vi "Mode 3.vi"() -> ()   [LabVIEW 2020]
uses:
  <vilib>/MakerHub/LINX/Private/Device/Type Defs/Pulse Polarity.ctl
  <vilib>/Platform/TimedLoop/XDataNode/timing_clust.ctl
  <vilib>/Platform/TimedLoop/XDataNode/nitl_modes.ctl
  <vilib>/Platform/TimedLoop/XDataNode/wakeup.ctl
  <vilib>/MakerHub/LINX/Public/Peripherals/Digital/Digital Write N Chans.vi
  <vilib>/MakerHub/LINX/Public/Peripherals/Digital/Digital Read N Chans.vi
  <vilib>/MakerHub/LINX/Public/Peripherals/PWM/PWM Set Duty Cycle 1 Chan.vi
  <vilib>/MakerHub/LINX/Private/Local IO/LinxDigitalWrite.vi
  <vilib>/MakerHub/LINX/Public/Utilities/Check Channel.vi
  <vilib>/MakerHub/LINX/Private/Local IO/LinxDigitalRead.vi
  <vilib>/MakerHub/LINX/Public/Utilities/Open Serial.vi
  <vilib>/MakerHub/LINX/Private/Utilties/Generate Error.vi
  <vilib>/MakerHub/LINX/Public/Sensors/Motion/Servo/Servo Open N Channels.vi
  <vilib>/MakerHub/LINX/Public/Sensors/Motion/Servo/Servo Set Pulse Width One Channel.vi
  <vilib>/MakerHub/LINX/Public/Peripherals/PWM/PWM Set Duty Cycle N Chans.vi
  <vilib>/MakerHub/LINX/Public/Sensors/Motion/Servo/Servo Close N Channels.vi
  <vilib>/platform/TimedLoop/XDataNode/XDataNode.xnode
  <vilib>/MakerHub/LINX/LMH-LINX.lvlib
  <vilib>/Platform/TimedLoop/XDataNode/XDNodeRunTimeDep.lvlib
  <vilib>/MakerHub/LINX/Public/Sensors/Motion/Servo/Servo.lvlib
  <vilib>/MakerHub/LINX/Private/Device/Device.lvlib
panel:
  in  "Titik Stop":u16=115
  in  "Color Check?":bool
  out "Blue Freq":u32
  out "Green Freq":u32
  out "Red Freq":u32
  out "Blue Workpiece":bool
  in  "Values":bool[](array[boolean])
  in  "Servo Slider 2 Angle":u16(knob)=82 scale=0.0..180.0
  in  "Servo Slider 1 Angle":u16(knob)=84 scale=0.0..180.0
  in  "Servo Magazine Angle":u16(knob)=115 scale=0.0..180.0
  in  "Servo Slider 2":u8=4
  in  "Servo Slider 1":u8=5
  in  "Servo Magazine":u8=3
  in  "Slider Counter":dbl[](array[numeric])=[0.0, 0.0, 0.0, 13.0]
  out "Green Workpiece":bool
  out "Red Workpiece":bool
  in  "Main Program":T1(array[cluster])=[{"Mode"=enum."Idle", "Limit"=enum."Tidak Ada", "Delay"=1000, "Point"=0, "Row"=0}, {"Mode"=enum."Cek Ketersediaan", "Limit"=enum."Tidak Ada", "Delay"=500, "Point"=0, "Row"=1}, {"Mode"=enum."Workpiece Masuk", "Limit"=enum."Tidak Ada", "Delay"=0, "Point"=0, "Row"=2}, {"Mode"=enum."Cek Warna", "Limit"=enum."Tidak Ada", "Delay"=1000, "Point"=0, "Row"=3}, {"Mode"=enum."Cek Counter", "Limit"=enum."Tidak Ada", "Delay"=1000, "Point"=0, "Row"=4}, {"Mode"=enum."Servo Set", "Limit"=enum."Tidak Ada", "Delay"=1000, "Point"=0, "Row"=5}, {"Mode"=enum."Conveyor Jalan", "Limit"=enum."Tidak Ada", "Delay"=0, "Point"=0, "Row"=6}, {"Mode"=enum."Servo Reset", "Limit"=enum."Tidak Ada", "Delay"=1000, "Point"=0, "Row"=7}, {"Mode"=enum."Counter", "Limit"=enum."Tidak Ada", "Delay"=0, "Point"=0, "Row"=8}, {"Mode"=enum."Go To", "Limit"=enum."Tidak Ada", "Delay"=0, "Point"=1, "Row"=9}]
  in  "Stop Main Program":bool
  out "Row":i32
  in  "Start Main Program":bool
  in  "Check Point":i32
  in  "STOP":bool
  in  "Speed Pin":u8=2
  in  "Sensors Pin":u8[](array[numeric])=[30, 34, 36, 38, 36, 38]
  out "Sensor Value":bool[](array[boolean])
  in  "Duty Cycle":dbl(knob) scale=0.0..100.0
  out "Device Name":string
  in  "Arduino Port":refnum<visa-resource-name>="N/A"
  # "LOW COST MPS SORTING BASED ARDUINO"
  # "MAIN PROGRAM"
  # "PROJECT MONITOR"
  # "Slider 1"
  # "Slider 2"
  # "Slider 3"
  # "INPUT/OUTPUT CONTROL"
  # "Index Array Sensors Pin\n\n0. IR Sensor Stock Check\n1. IR Sensor Slider 1\n2. IR Sensor Slider 2\n3. IR Sensor Slider 3"
  # "Mechatronics Engineering 2nd Generation - Vocational High School 2 Bojonegoro"
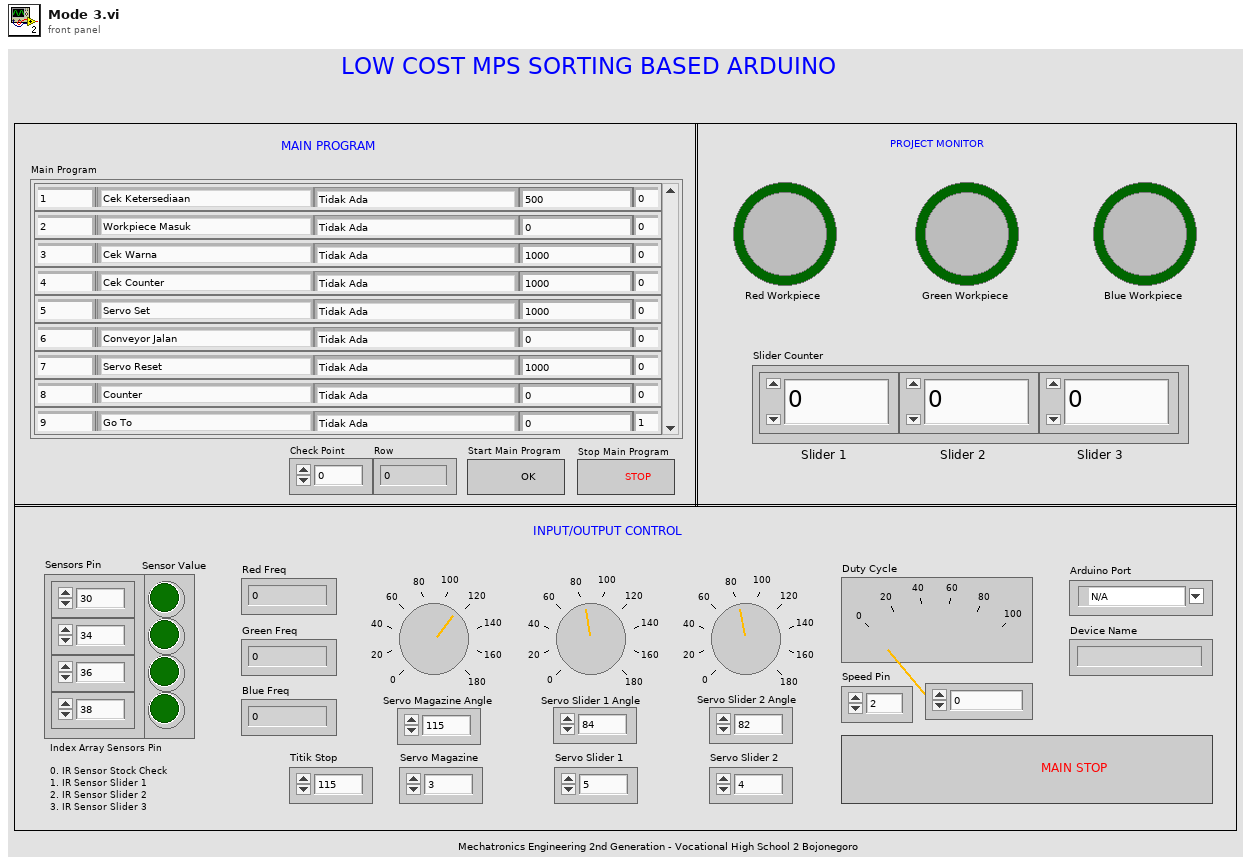
[diagram p1: front panel]
types:
  T1 = cluster{"Mode":enum16{"Idle", "Cek Ketersediaan", "Workpiece Masuk", "Cek Warna", "Servo Set", "Conveyor Jalan", "Servo Reset", "Counter", "Cek Counter", "Go To"}, "Limit":enum16{"Tidak Ada", "Sensor Slider"}, "Delay":i32, "Point":i32, "Row":i32}[]
  T2 = typedef "XDNodeRunTimeDep.lvlib/timing_clust.ctl" = cluster{"Expected End [f-1]":u64, "Actual End [f-1]":u64, "Finished Late? [f-1]":bool, "Expected End [i-1]":u64, "Actual End [i-1]":u64, "Finished Late? [i-1]":bool, "Expected Start [i]":u64, "Actual Start [i]":u64, "Expected Start [f]":u64, "Actual Start [f]":u64, "Source Name":string, "Structure Name":string, "Period":i64, "Deadline":i64, "Offset":i64, "Start":i64, "Priority":i32, "Timeout":i32, "Mode":T3, "Wakeup Reason":T4, "Error":errorcluster, "Source Type":string, "Secondary Source Type":string, "Global End Time":u64, "Global Start Time":u64, "Frame Duration":u64, "Iteration Duration":u64, "Assigned CPU":i32, "I/O Scan Engine Mode":u32}
  T3 = typedef "XDNodeRunTimeDep.lvlib/nitl_modes.ctl" = enum32{"No Change", "Process missed periods, maintain original phase", "Discard missed periods, maintain original phase", "Process missed periods, ignore original phase", "Discard missed periods, ignore original phase"}
  T4 = typedef "XDNodeRunTimeDep.lvlib/wakeup.ctl" = enum32{"Normal", "Aborted", "Asynchronous wakeup", "Timing source error", "Timed loop error", "Timeout"}
  T5 = cluster{"Mode":enum16{"Idle", "Cek Ketersediaan", "Workpiece Masuk", "Cek Warna", "Servo Set", "Conveyor Jalan", "Servo Reset", "Counter", "Cek Counter", "Go To"}, "Limit":enum16{"Tidak Ada", "Sensor Slider"}, "Delay":i32, "Point":i32, "Row":i32}
  T6 = enum16{"Idle", "Cek Ketersediaan", "Workpiece Masuk", "Cek Warna", "Servo Set", "Conveyor Jalan", "Servo Reset", "Counter", "Cek Counter", "Go To"}
  T7 = typedef "LMH-LINX.lvlib/LINX Ref.ctl" = cluster{"IO":T8, "Interface":T9, "LINX Device Config":T10}
  T8 = typedef "LMH-LINX.lvlib/Platform.ctl" = enum16{"Remote", "Local"}
  T9 = typedef "LMH-LINX.lvlib/Interface.ctl" = enum16{"Serial", "TCP"}
  T10 = typedef "LMH-LINX.lvlib/Device.lvlib/LINX Device Config.ctl" = cluster{"Interface":T9, "COM Port":refnum<visa-resource-name>, "TCP Configuration":T11, "Device Family":u8, "Device ID":u8, "Device Name":string, "TCP Ref":refnum<k5>, "Channels":T12}
  T11 = typedef "LMH-LINX.lvlib/Device.lvlib/TCP Config.ctl" = cluster{"IP Address":string, "Port":u16}
  T12 = typedef "LMH-LINX.lvlib/Channels.ctl" = cluster{"DI":u8[], "DO":u8[], "AI":u8[], "AO":u8[], "PWM":u8[], "QE":u8[], "UART":u8[], "I2C 2":u8[], "SPI":u8[], "CAN":u8[], "Servo":u8[], "AI Ref (V)":dbl, "AI Resolution (Bits)":u8, "AO Ref (V)":dbl, "AO Resolution (Bits)":u8}
  T13 = typedef "LMH-LINX.lvlib/Device.lvlib/Pulse Polarity.ctl" = enum8{"Active Low", "Active High"}
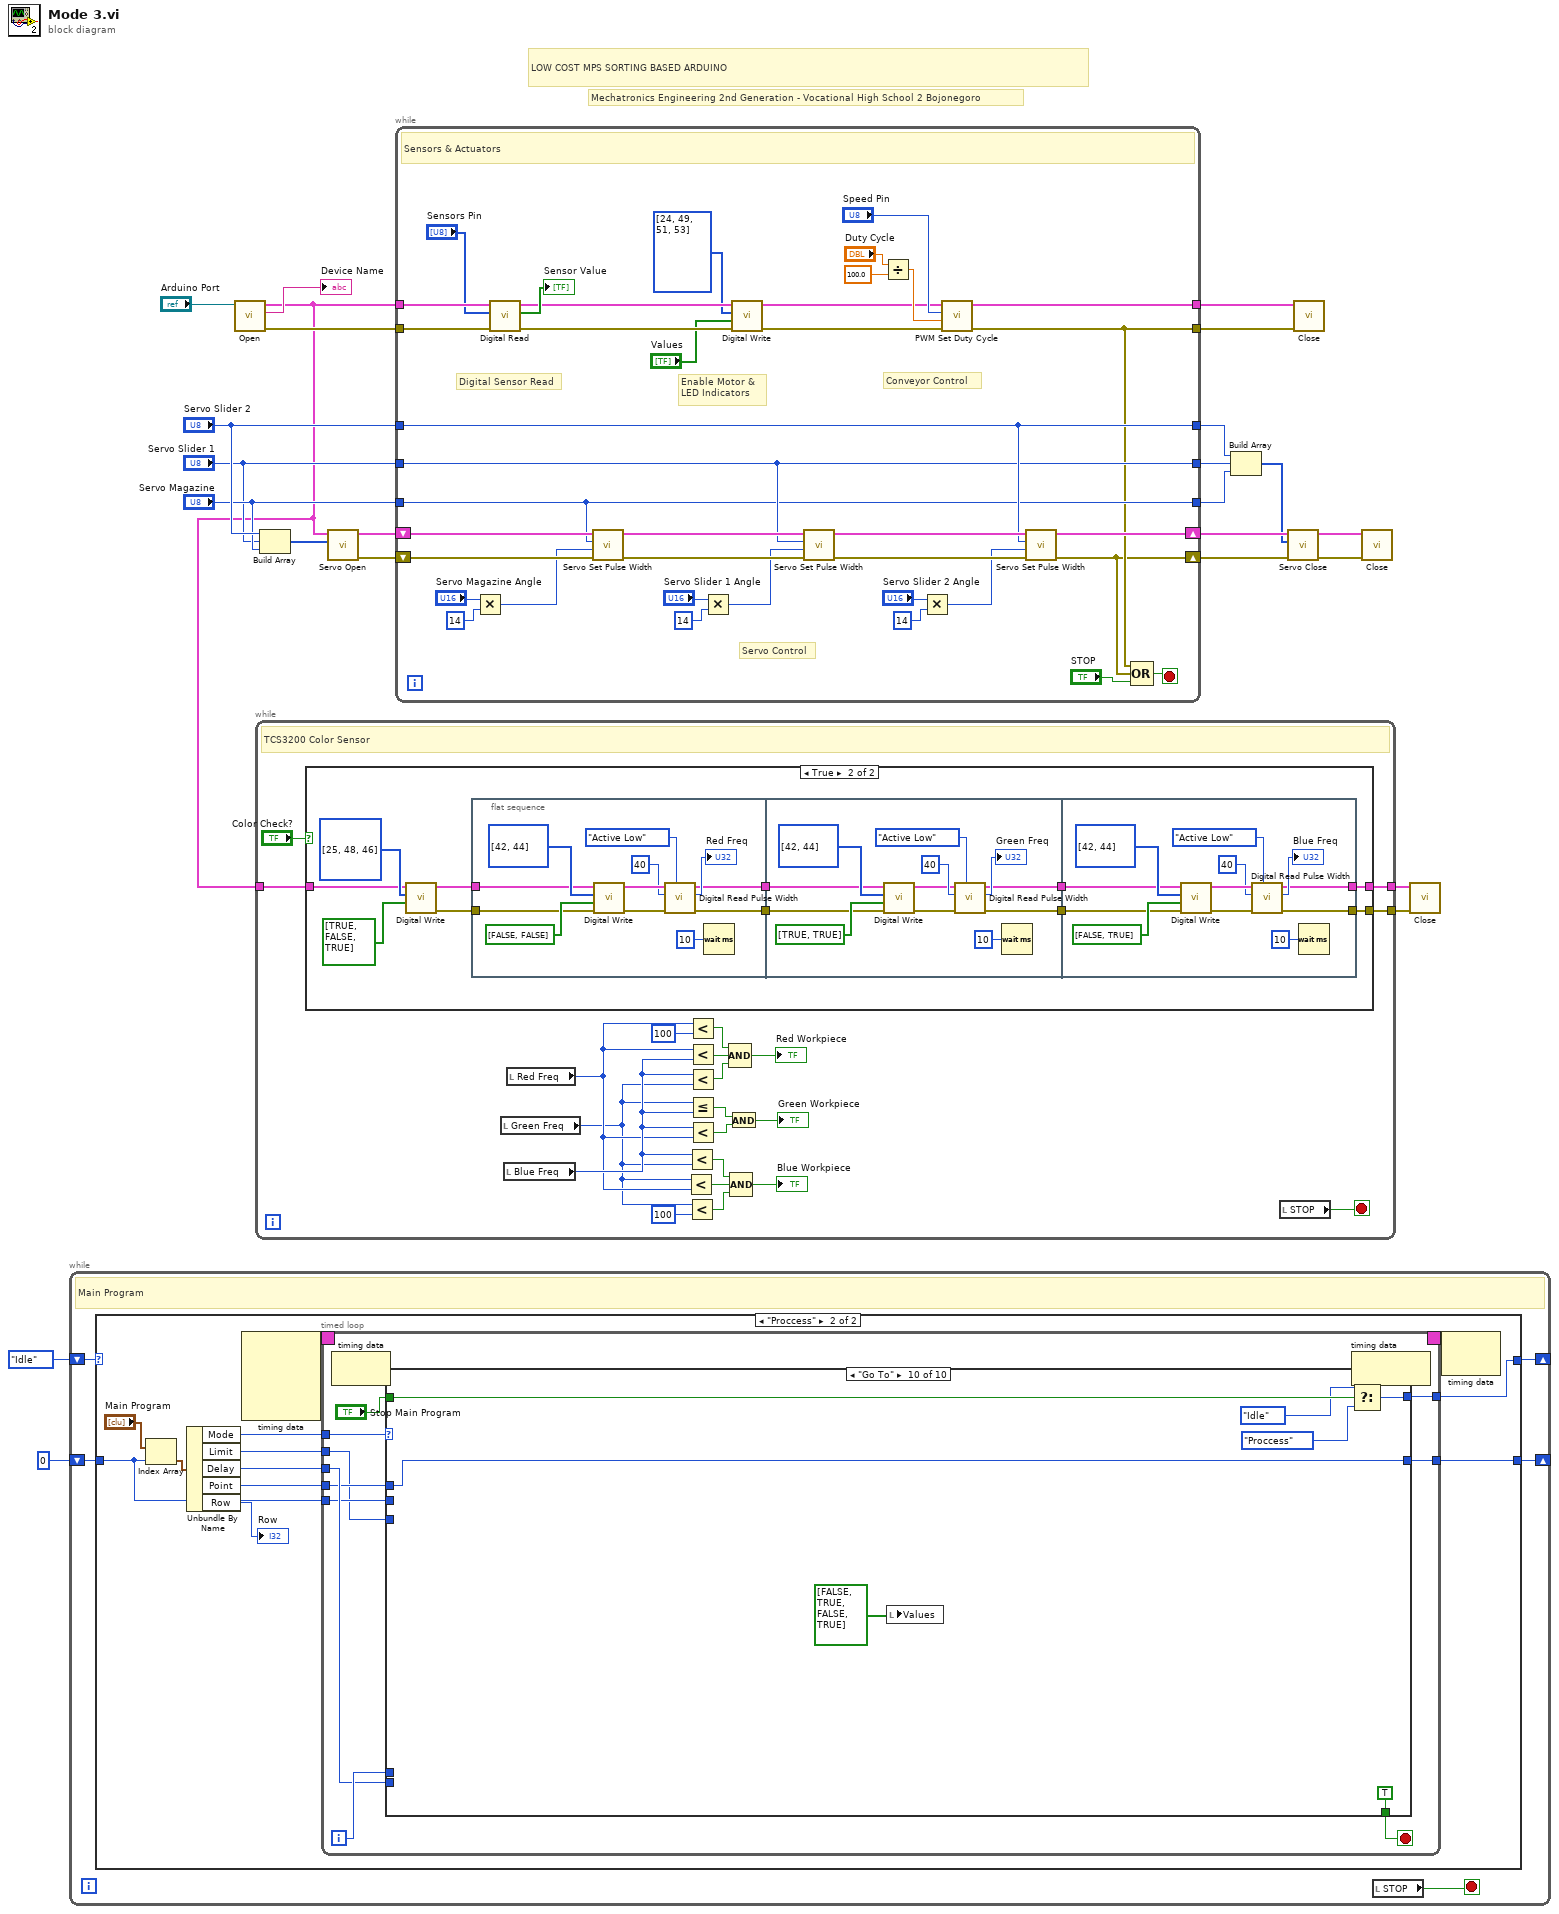
[diagram p0: block diagram]
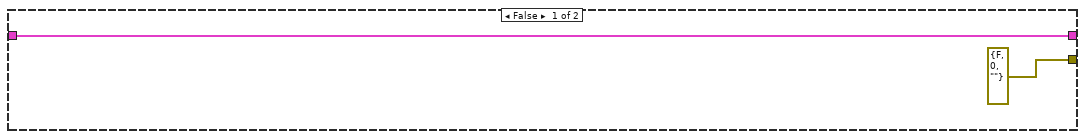
[diagram p2: hidden frame]
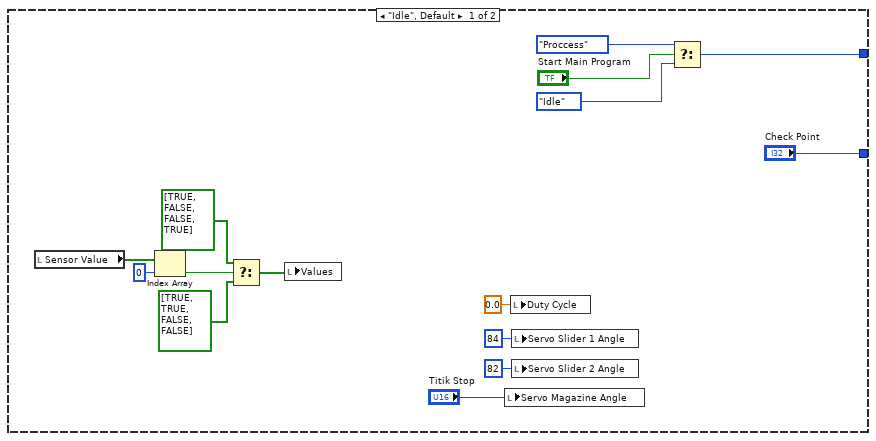
[diagram p3: hidden frame]
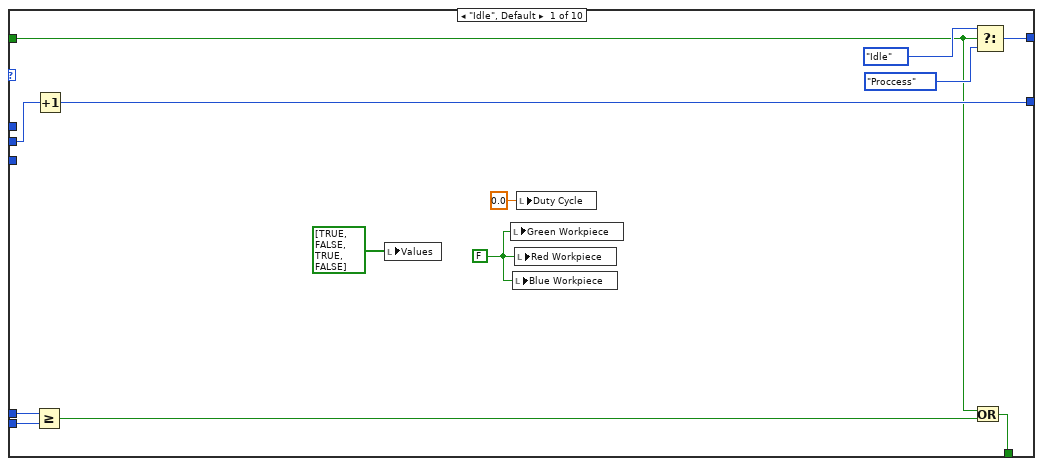
[diagram p4: hidden frame]
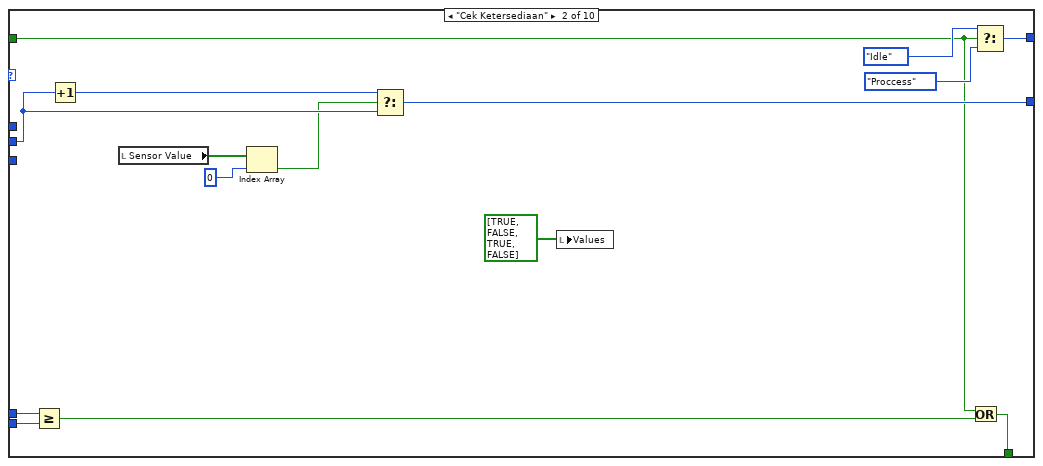
[diagram p5: hidden frame]
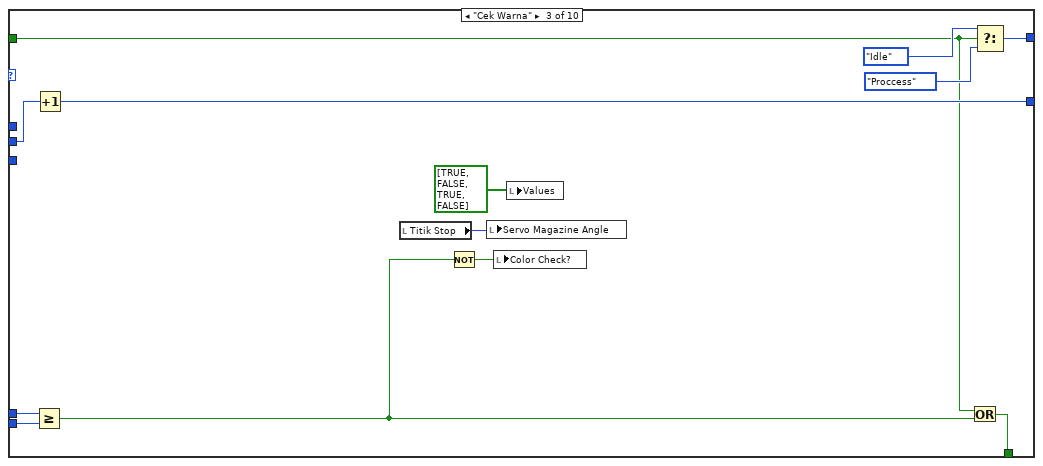
[diagram p6: hidden frame]
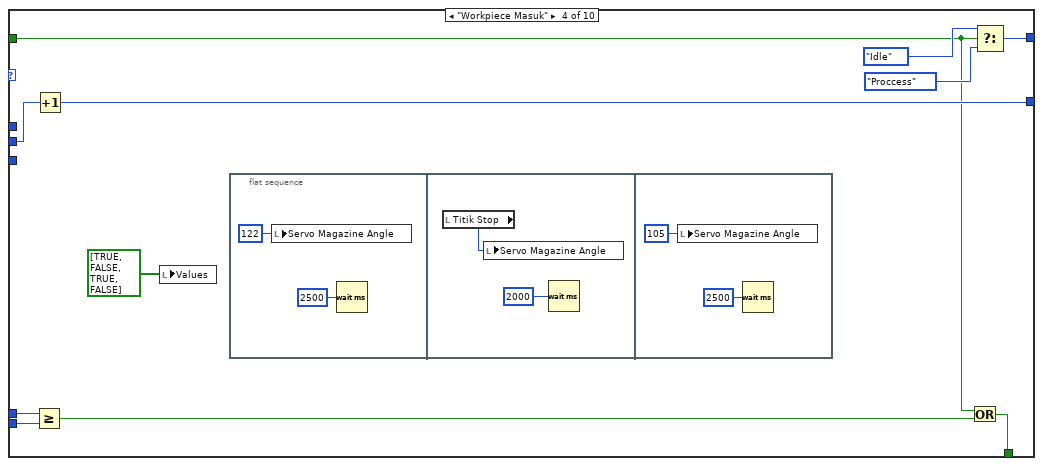
[diagram p7: hidden frame]
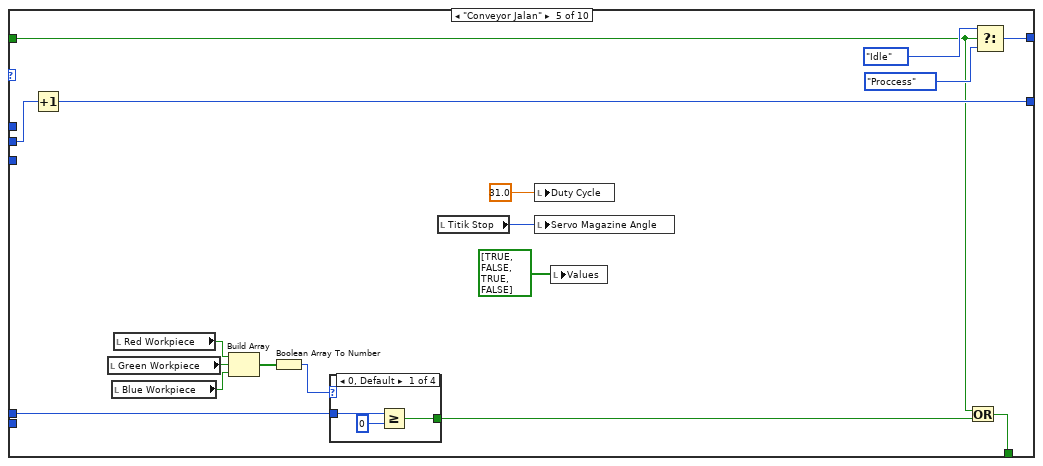
[diagram p8: hidden frame]
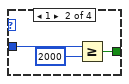
[diagram p9: hidden frame]
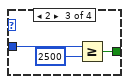
[diagram p10: hidden frame]
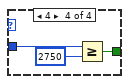
[diagram p11: hidden frame]
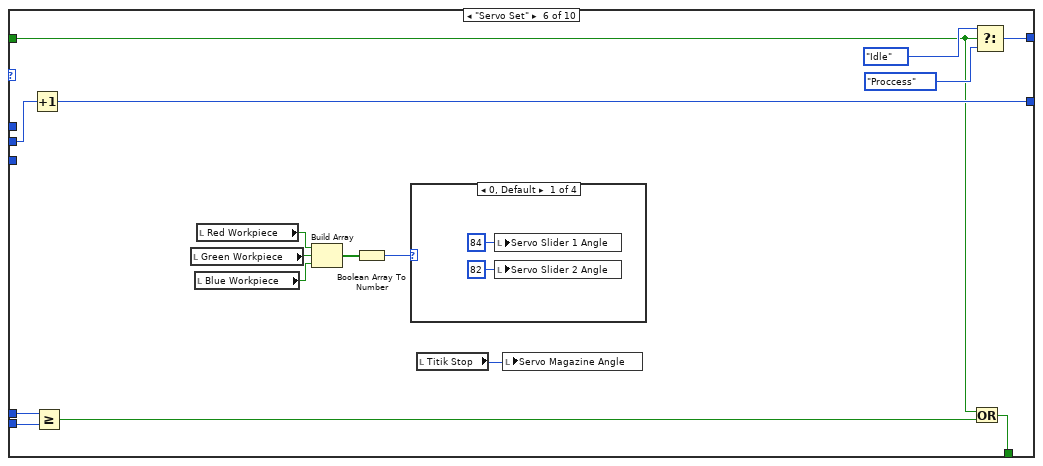
[diagram p12: hidden frame]
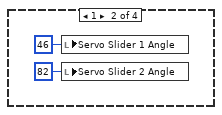
[diagram p13: hidden frame]
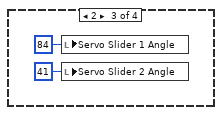
[diagram p14: hidden frame]
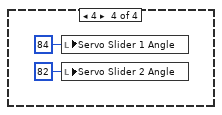
[diagram p15: hidden frame]
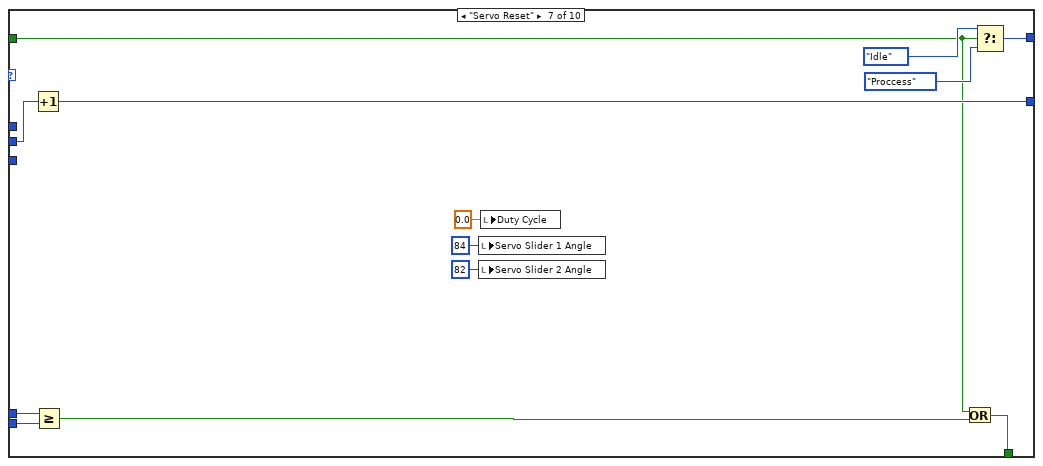
[diagram p16: hidden frame]
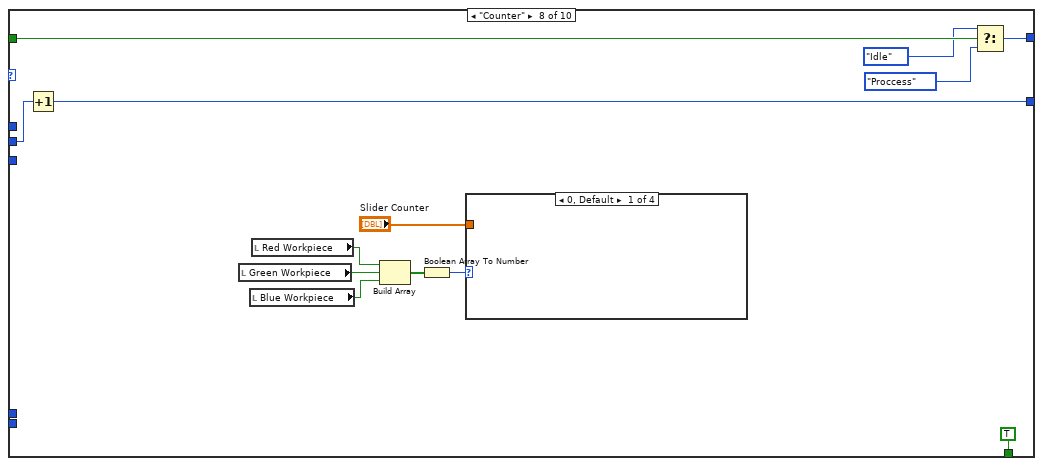
[diagram p17: hidden frame]
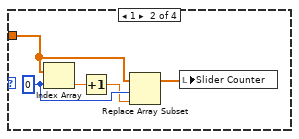
[diagram p18: hidden frame]
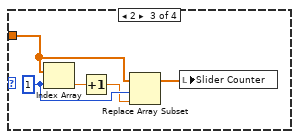
[diagram p19: hidden frame]
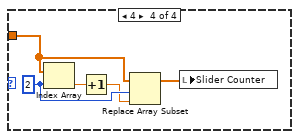
[diagram p20: hidden frame]
diagram:
  # "Mechatronics Engineering 2nd Generation - Vocational High School 2 Bojonegoro"
  # "LOW COST MPS SORTING BASED ARDUINO"
  n1 = while {
    shift-right: [w27] -> _
    shift-left: enum16{"Idle", "Proccess"}."Idle" -> [w28]
    shift-right: [w25] -> _
    shift-left: 0 ("index") -> [w26]
    stop <- w29 stop-if-true
    # "Main Program"
    n2 = case shown="\"Proccess\"" w28 {
      tunnel: [w44 w53] -> w27
      tunnel: w26 -> [_ w52]
      tunnel: ["Check Point" w51] -> w25
      frame "Idle", Default {
        n3 = local read "Sensor Value"() -> (w36:bool[])
        n4 = Index Array(array=w36, index=0) -> (element=w34:bool)
        n5 = Select(t=bool[] [TRUE, FALSE, FALSE, TRUE] ("Values"), s=w34, f=bool[] [TRUE, TRUE, FALSE, FALSE] ("Values")) -> (s? t:f=w31:bool[])
        n6 = local write "Values"(w31) -> ()
        n7 = local write "Servo Magazine Angle"("Titik Stop") -> ()
        n8 = local write "Duty Cycle"(0.0 ("Duty Cycle")) -> ()
        n9 = local write "Servo Slider 1 Angle"(u16 84 ("Servo Slider 1 Angle")) -> ()
        n10 = local write "Servo Slider 2 Angle"(u16 82 ("Servo Slider 2 Angle")) -> ()
        n11 = Select(t=enum16{"Idle", "Proccess"}."Proccess", s="Start Main Program", f=enum16{"Idle", "Proccess"}."Idle") -> (s? t:f=w44:enum16{"Idle", "Proccess"})
      }
      frame "Proccess" {
        n12 = Index Array(array="Main Program", index=w52) -> (element=w56:T5)
        n13 = Unbundle By Name(w56) -> ("Mode"=w55:T6, "Limit"=w47:enum16{"Tidak Ada", "Sensor Slider"}, "Delay"=w54:i32, "Point"=w48:i32, "Row"=→"Row":i32)
        n14 = node-c288() -> (w50:T2)  [unwired: 4 in]
        n15 = timed-loop {
          tunnel: w55 -> [w66]
          tunnel: w54 -> [w64]
          tunnel: [w62] -> w53
          tunnel: w52 -> [w61]
          tunnel: [w60] -> w51
          timing: w50 -> [_]
          timing-out: [_] -> w49
          tunnel: w48 -> [w59]
          tunnel: w47 -> [w58]
          i -> [w65]
          stop <- w63 stop-if-true
          n16 = node-c288() -> ()  [unwired: 1 in, 1 out]
          n17 = case shown="\"Go To\"" w66 {
            tunnel: w65 -> [w75 w92 w105 w114 w131 w166 w187 _ _ _]
            tunnel: w64 -> [w76 w93 w106 w115 _ w165 w186 _ _ _]
            tunnel: [w71 w84 w99 w112 w129 w157 w182 TRUE TRUE TRUE] -> w63
            tunnel: "Stop Main Program" -> [w70 w83 w100 w111 w128 w158 w181 w204 w227 w258]
            tunnel: [w81 w96 w109 w120 w143 w171 w192 w205 w236 w259] -> w62
            tunnel: w61 -> [w78 w87 w104 w117 w139 w168 w189 w201 w233 _]
            tunnel: [w77 w89 w103 w116 w140 w167 w188 w200 w232 w255] -> w60
            tunnel: w59 -> [_ _ _ _ _ _ _ _ _ w255]
            tunnel: w58 -> [_ _ _ _ _ _ _ _ _ _]
            frame "Idle", Default {
              w74 = FALSE ("Benda Hijau")
              n18 = Greater Or Equal?(x=w75, y=w76) -> (x >= y?=w69:bool)
              n19 = Increment(x=w78) -> (x+1=w77:i32)
              n20 = local write "Values"(bool[] [TRUE, FALSE, TRUE, FALSE] ("Values")) -> ()
              n21 = local write "Green Workpiece"(w74) -> ()
              n22 = local write "Blue Workpiece"(w74) -> ()
              n23 = local write "Red Workpiece"(w74) -> ()
              n24 = local write "Duty Cycle"(0.0 ("Duty Cycle")) -> ()
              n25 = Or(x=w70, y=w69) -> (x .or. y?=w71:bool)
              n26 = Select(t=enum16{"Idle", "Proccess"}."Idle", s=w70, f=enum16{"Idle", "Proccess"}."Proccess") -> (s? t:f=w81:enum16{"Idle", "Proccess"})
            }
            frame "Cek Ketersediaan" {
              n27 = Greater Or Equal?(x=w92, y=w93) -> (x >= y?=w82:bool)
              n28 = Increment(x=w87) -> (x+1=w88:i32)
              n29 = local read "Sensor Value"() -> (w91:bool[])
              n30 = Index Array(array=w91, index=0) -> (element=w86:bool)
              n31 = Select(t=w88, s=w86, f=w87) -> (s? t:f=w89:i32)
              n32 = local write "Values"(bool[] [TRUE, FALSE, TRUE, FALSE] ("Values")) -> ()
              n33 = Or(x=w83, y=w82) -> (x .or. y?=w84:bool)
              n34 = Select(t=enum16{"Idle", "Proccess"}."Idle", s=w83, f=enum16{"Idle", "Proccess"}."Proccess") -> (s? t:f=w96:enum16{"Idle", "Proccess"})
            }
            frame "Cek Warna" {
              n35 = Greater Or Equal?(x=w105, y=w106) -> (x >= y?=w97:bool)
              n36 = Increment(x=w104) -> (x+1=w103:i32)
              n37 = local read "Titik Stop"() -> (w101:u16)
              n38 = Not(x=w97) -> (.not. x?=w98:bool)
              n39 = local write "Servo Magazine Angle"(w101) -> ()
              n40 = local write "Color Check?"(w98) -> ()
              n41 = local write "Values"(bool[] [TRUE, FALSE, TRUE, FALSE] ("Values")) -> ()
              n42 = Or(x=w100, y=w97) -> (x .or. y?=w99:bool)
              n43 = Select(t=enum16{"Idle", "Proccess"}."Idle", s=w100, f=enum16{"Idle", "Proccess"}."Proccess") -> (s? t:f=w109:enum16{"Idle", "Proccess"})
            }
            frame "Workpiece Masuk" {
              n44 = Greater Or Equal?(x=w114, y=w115) -> (x >= y?=w110:bool)
              n45 = Increment(x=w117) -> (x+1=w116:i32)
              n46 = local write "Values"(bool[] [TRUE, FALSE, TRUE, FALSE] ("Values")) -> ()
              n47 = flat-sequence {
                frame #0 {
                  n48 = local write "Servo Magazine Angle"(u16 122 ("Servo Magazine Angle")) -> ()
                  n49 = Wait (ms)(milliseconds to wait=u32 2500) -> ()  [unwired: 1 out]
                }
                frame #1 {
                  n50 = local read "Titik Stop"() -> (w123:u16)
                  n51 = local write "Servo Magazine Angle"(w123) -> ()
                  n52 = Wait (ms)(milliseconds to wait=u32 2000) -> ()  [unwired: 1 out]
                }
                frame #2 {
                  n53 = local write "Servo Magazine Angle"(u16 105 ("Servo Magazine Angle")) -> ()
                  n54 = Wait (ms)(milliseconds to wait=u32 2500) -> ()  [unwired: 1 out]
                }
              }
              n55 = Or(x=w111, y=w110) -> (x .or. y?=w112:bool)
              n56 = Select(t=enum16{"Idle", "Proccess"}."Idle", s=w111, f=enum16{"Idle", "Proccess"}."Proccess") -> (s? t:f=w120:enum16{"Idle", "Proccess"})
            }
            frame "Conveyor Jalan" {
              n57 = Increment(x=w139) -> (x+1=w140:i32)
              n58 = local read "Green Workpiece"() -> (w135:bool)
              n59 = local read "Blue Workpiece"() -> (w134:bool)
              n60 = local read "Red Workpiece"() -> (w136:bool)
              n61 = Build Array(w136, w135, w134) -> (w133:bool[])
              n62 = Boolean Array To Number(Boolean array=w133) -> (number=w132:u32)
              n63 = case shown="0, Default" w132 {
                tunnel: [w146 w149 w152 w155] -> w127
                tunnel: w131 -> [w145 w148 w151 w154]
                frame 0, Default {
                  n64 = Greater Or Equal?(x=w145, y=0) -> (x >= y?=w146:bool)
                }
                frame 1 {
                  n65 = Greater Or Equal?(x=w148, y=2000) -> (x >= y?=w149:bool)
                }
                frame 2 {
                  n66 = Greater Or Equal?(x=w151, y=2500) -> (x >= y?=w152:bool)
                }
                frame 4 {
                  n67 = Greater Or Equal?(x=w154, y=2750) -> (x >= y?=w155:bool)
                }
              }
              n68 = local read "Titik Stop"() -> (w130:u16)
              n69 = local write "Duty Cycle"(31.0 ("Duty Cycle (0-1)")) -> ()
              n70 = local write "Servo Magazine Angle"(w130) -> ()
              n71 = local write "Values"(bool[] [TRUE, FALSE, TRUE, FALSE] ("Values")) -> ()
              n72 = Or(x=w128, y=w127) -> (x .or. y?=w129:bool)
              n73 = Select(t=enum16{"Idle", "Proccess"}."Idle", s=w128, f=enum16{"Idle", "Proccess"}."Proccess") -> (s? t:f=w143:enum16{"Idle", "Proccess"})
            }
            frame "Servo Set" {
              n74 = Increment(x=w168) -> (x+1=w167:i32)
              n75 = Greater Or Equal?(x=w166, y=w165) -> (x >= y?=w156:bool)
              n76 = local read "Green Workpiece"() -> (w163:bool)
              n77 = local read "Blue Workpiece"() -> (w162:bool)
              n78 = local read "Red Workpiece"() -> (w164:bool)
              n79 = Build Array(w164, w163, w162) -> (w161:bool[])
              n80 = Boolean Array To Number(Boolean array=w161) -> (number=w160:u32)
              n81 = case shown="0, Default" w160 {
                frame 0, Default {
                  n82 = local write "Servo Slider 1 Angle"(u16 84 ("Servo Slider 1 Angle")) -> ()
                  n83 = local write "Servo Slider 2 Angle"(u16 82 ("Servo Slider 2 Angle")) -> ()
                }
                frame 1 {
                  n84 = local write "Servo Slider 1 Angle"(u16 46 ("Servo Slider 1 Angle")) -> ()
                  n85 = local write "Servo Slider 2 Angle"(u16 82 ("Servo Slider 2 Angle")) -> ()
                }
                frame 2 {
                  n86 = local write "Servo Slider 1 Angle"(u16 84 ("Servo Slider 1 Angle")) -> ()
                  n87 = local write "Servo Slider 2 Angle"(u16 41 ("Servo Slider 2 Angle")) -> ()
                }
                frame 4 {
                  n88 = local write "Servo Slider 1 Angle"(u16 84 ("Servo Slider 1 Angle")) -> ()
                  n89 = local write "Servo Slider 2 Angle"(u16 82 ("Servo Slider 2 Angle")) -> ()
                }
              }
              n90 = local read "Titik Stop"() -> (w159:u16)
              n91 = local write "Servo Magazine Angle"(w159) -> ()
              n92 = Or(x=w158, y=w156) -> (x .or. y?=w157:bool)
              n93 = Select(t=enum16{"Idle", "Proccess"}."Idle", s=w158, f=enum16{"Idle", "Proccess"}."Proccess") -> (s? t:f=w171:enum16{"Idle", "Proccess"})
            }
            frame "Servo Reset" {
              n94 = Increment(x=w189) -> (x+1=w188:i32)
              n95 = Greater Or Equal?(x=w187, y=w186) -> (x >= y?=w180:bool)
              n96 = local write "Servo Slider 1 Angle"(u16 84 ("Servo Slider 1 Angle")) -> ()
              n97 = local write "Servo Slider 2 Angle"(u16 82 ("Servo Slider 2 Angle")) -> ()
              n98 = local write "Duty Cycle"(0.0 ("Duty Cycle")) -> ()
              n99 = Or(x=w181, y=w180) -> (x .or. y?=w182:bool)
              n100 = Select(t=enum16{"Idle", "Proccess"}."Idle", s=w181, f=enum16{"Idle", "Proccess"}."Proccess") -> (s? t:f=w192:enum16{"Idle", "Proccess"})
            }
            frame "Counter" {
              n101 = Increment(x=w201) -> (x+1=w200:i32)
              n102 = local read "Green Workpiece"() -> (w194:bool)
              n103 = local read "Blue Workpiece"() -> (w193:bool)
              n104 = local read "Red Workpiece"() -> (w195:bool)
              n105 = Build Array(w195, w194, w193) -> (w198:bool[])
              n106 = Boolean Array To Number(Boolean array=w198) -> (number=w197:u32)
              n107 = case shown="0, Default" w197 {
                tunnel: "Slider Counter" -> [_ w206 w211 w216]
                frame 0, Default {
                }
                frame 1 {
                  w208 = 0 ("index")
                  n108 = Index Array(array=w206, index=w208) -> (element=w210:dbl)
                  n109 = Increment(x=w210) -> (x+1=w207:dbl)
                  n110 = Replace Array Subset(array=w206, new element=w207, index=w208) -> (w209:dbl[])
                  n111 = local write "Slider Counter"(w209) -> ()
                }
                frame 2 {
                  w213 = 1 ("index")
                  n112 = Index Array(array=w211, index=w213) -> (element=w215:dbl)
                  n113 = Increment(x=w215) -> (x+1=w212:dbl)
                  n114 = Replace Array Subset(array=w211, new element=w212, index=w213) -> (w214:dbl[])
                  n115 = local write "Slider Counter"(w214) -> ()
                }
                frame 4 {
                  w218 = 2 ("index")
                  n116 = Index Array(array=w216, index=w218) -> (element=w220:dbl)
                  n117 = Increment(x=w220) -> (x+1=w217:dbl)
                  n118 = Replace Array Subset(array=w216, new element=w217, index=w218) -> (w219:dbl[])
                  n119 = local write "Slider Counter"(w219) -> ()
                }
              }
              n120 = Select(t=enum16{"Idle", "Proccess"}."Idle", s=w204, f=enum16{"Idle", "Proccess"}."Proccess") -> (s? t:f=w205:enum16{"Idle", "Proccess"})
            }
            frame "Cek Counter" {
              n121 = Increment(x=w233) -> (x+1=w232:i32)
              n122 = local read "Green Workpiece"() -> (w225:bool)
              n123 = local read "Blue Workpiece"() -> (w223:bool)
              n124 = local read "Red Workpiece"() -> (w224:bool)
              n125 = local read "Slider Counter"() -> (w229:dbl[])
              n126 = Build Array(w224, w225, w223) -> (w222:bool[])
              n127 = Boolean Array To Number(Boolean array=w222) -> (number=w230:u32)
              n128 = local write "Color Check?"(FALSE ("Cek Warna?")) -> ()
              n129 = case shown="0, Default" w230 {
                tunnel: w229 -> [_ w241 w246 w251]
                tunnel: [FALSE w238 w243 w248] -> w226
                frame 0, Default {
                }
                frame 1 {
                  n130 = Index Array(array=w241, index=0) -> (element=w240:dbl)
                  n131 = Greater Or Equal?(x=w240, y=3.0) -> (x >= y?=w238:bool)
                }
                frame 2 {
                  n132 = Index Array(array=w246, index=1) -> (element=w245:dbl)
                  n133 = Greater Or Equal?(x=w245, y=3.0) -> (x >= y?=w243:bool)
                }
                frame 4 {
                  n134 = Index Array(array=w251, index=2) -> (element=w250:dbl)
                  n135 = Greater Or Equal?(x=w250, y=3.0) -> (x >= y?=w248:bool)
                }
              }
              n136 = Or(x=w227, y=w226) -> (x .or. y?=w228:bool)
              n137 = Select(t=enum16{"Idle", "Proccess"}."Idle", s=w228, f=enum16{"Idle", "Proccess"}."Proccess") -> (s? t:f=w236:enum16{"Idle", "Proccess"})
            }
            frame "Go To" {
              n138 = local write "Values"(bool[] [FALSE, TRUE, FALSE, TRUE] ("Values")) -> ()
              n139 = Select(t=enum16{"Idle", "Proccess"}."Idle", s=w258, f=enum16{"Idle", "Proccess"}."Proccess") -> (s? t:f=w259:enum16{"Idle", "Proccess"})
            }
          }
          n140 = node-c288() -> ()  [unwired: 1 in, 1 out]
        }
        n141 = node-c288(w49) -> ()  [unwired: 1 out]
      }
    }
    n142 = local read "STOP"() -> (w29:bool)
  }
  n143 = call-poly <vilib>:"Open.vi"("Serial Port"="Arduino Port") -> ("Error Out"=w22:errorcluster, "Device Name"=→"Device Name":string, "LINX Resource"=w1:T7)  [unwired: 8 in]
  n144 = while {
    tunnel: [w282] -> w3
    tunnel: [w281] -> w2
    tunnel: w1 -> [w262]
    stop <- w264 stop-if-true
    # "TCS3200 Color Sensor"
    n145 = case shown="True" "Color Check?" {
      tunnel: w262 -> [w284 w285]
      tunnel: [w284 w291] -> w282
      tunnel: [errorcluster {"status"=FALSE, "code"=0, "source"=""} ("Error Out") w290] -> w281
      frame False {
      }
      frame True {
        n146 = call-poly <vilib>:"Digital Write.vi"("Values"=bool[] [TRUE, FALSE, TRUE], "DO Channels"=u8[] [25, 48, 46], "LINX Resource"=w285) -> ("Error Out"=w286:errorcluster, "LINX Resource"=w287:T7)  [unwired: 7 in]
        n147 = flat-sequence {
          tunnel: w287 -> [w303]
          tunnel: w286 -> [w302]
          tunnel: [w298] -> w295
          tunnel: [w297] -> w294
          tunnel: w295 -> [w312]
          tunnel: w294 -> [w311]
          tunnel: [w309] -> w293
          tunnel: [w308] -> w292
          tunnel: w293 -> [w323]
          tunnel: w292 -> [w322]
          tunnel: [w321] -> w291
          tunnel: [w320] -> w290
          frame #0 {
            n148 = call-poly <vilib>:"Digital Write.vi"("Error In"=w302, "Values"=bool[] [FALSE, FALSE], "DO Channels"=u8[] [42, 44], "LINX Resource"=w303) -> ("Error Out"=w301:errorcluster, "LINX Resource"=w304:T7)  [unwired: 6 in]
            n149 = call <vilib>:"Digital Read Pulse Width.vi"("Incoming Pulse Polarity (Active High)"=Pulse_Polarity."Active Low", "Error In"=w301, "DI Channel"=u8 40, "LINX Resource"=w304) -> ("Error Out"=w297:errorcluster, "Pulse Width (uS)"=→"Red Freq":u32, "LINX Resource"=w298:T7)  [unwired: 5 in]
            n150 = Wait (ms)(milliseconds to wait=u32 10) -> ()  [unwired: 1 out]
          }
          frame #1 {
            n151 = call-poly <vilib>:"Digital Write.vi"("Error In"=w311, "Values"=bool[] [TRUE, TRUE], "DO Channels"=u8[] [42, 44], "LINX Resource"=w312) -> ("Error Out"=w317:errorcluster, "LINX Resource"=w316:T7)  [unwired: 6 in]
            n152 = call <vilib>:"Digital Read Pulse Width.vi"("Incoming Pulse Polarity (Active High)"=Pulse_Polarity."Active Low", "Error In"=w317, "DI Channel"=u8 40, "LINX Resource"=w316) -> ("Error Out"=w309:errorcluster, "Pulse Width (uS)"=→"Green Freq":u32, "LINX Resource"=w308:T7)  [unwired: 5 in]
            n153 = Wait (ms)(milliseconds to wait=u32 10) -> ()  [unwired: 1 out]
          }
          frame #2 {
            n154 = call-poly <vilib>:"Digital Write.vi"("Error In"=w323, "Values"=bool[] [FALSE, TRUE], "DO Channels"=u8[] [42, 44], "LINX Resource"=w322) -> ("Error Out"=w326:errorcluster, "LINX Resource"=w327:T7)  [unwired: 6 in]
            n155 = call <vilib>:"Digital Read Pulse Width.vi"("Incoming Pulse Polarity (Active High)"=Pulse_Polarity."Active Low", "Error In"=w326, "DI Channel"=u8 40, "LINX Resource"=w327) -> ("Error Out"=w320:errorcluster, "Pulse Width (uS)"=→"Blue Freq":u32, "LINX Resource"=w321:T7)  [unwired: 5 in]
            n156 = Wait (ms)(milliseconds to wait=u32 10) -> ()  [unwired: 1 out]
          }
        }
      }
    }
    n157 = local read "Green Freq"() -> (w275:u32)
    n158 = local read "Blue Freq"() -> (w277:u32)
    n159 = local read "Red Freq"() -> (w276:u32)
    n160 = Less?(x=w275, y=w276) -> (x < y?=w272:bool)
    n161 = Less?(x=w277, y=w275) -> (x < y?=w273:bool)
    n162 = Less?(x=w275, y=u32 100) -> (x < y?=w271:bool)
    n163 = Less?(x=w276, y=u32 100) -> (x < y?=w268:bool)
    n164 = Less?(x=w276, y=w277) -> (x < y?=w270:bool)
    n165 = Less?(x=w277, y=w275) -> (x < y?=w269:bool)
    n166 = Less Or Equal?(x=w275, y=w277) -> (x <= y?=w279:bool)
    n167 = Less?(x=w277, y=w276) -> (x < y?=w278:bool)
    n168 = Compound Arithmetic op=AND(w268, w270, w269) -> (→"Red Workpiece":bool)
    n169 = And(x=w279, y=w278) -> (x .and. y?=→"Green Workpiece":bool)
    n170 = Compound Arithmetic op=AND(w273, w272, w271) -> (→"Blue Workpiece":bool)
    n171 = local read "STOP"() -> (w264:bool)
  }
  n172 = Build Array("Servo Slider 2", "Servo Slider 1", "Servo Magazine") -> (w8:u8[])
  n173 = call-poly <vilib>:"Servo Open.vi"("Servo Channels"=w8, "LINX Resource"=w1) -> ("Error Out"=w18:errorcluster, "LINX Resource"=w19:T7)  [unwired: 8 in]
  n174 = while {
    tunnel: w1 -> [w367]
    tunnel: [w365] -> w24
    tunnel: [w337] -> w23
    tunnel: w22 -> [w366]
    shift-right: [w354] -> w12
    shift-left: w19 -> [w364]
    shift-right: [w336] -> w17
    shift-left: w18 -> [w363]
    tunnel: "Servo Magazine" -> [w355]
    tunnel: "Servo Slider 1" -> [w356]
    tunnel: "Servo Slider 2" -> [w357]
    tunnel: [w357] -> w6
    tunnel: [w356] -> w5
    tunnel: [w355] -> w4
    stop <- w369 stop-if-true
    # "Enable Motor &\nLED Indicators"
    # "Servo Control"
    # "Conveyor Control"
    # "Digital Sensor Read"
    # "Sensors & Actuators"
    n175 = Multiply(x="Servo Magazine Angle", y=u16 14) -> (x*y=w352:u16)
    n176 = call-poly <vilib>:"Digital Read.vi"("Error In"=w366, "DI Channels"="Sensors Pin", "LINX Resource"=w367) -> ("Error Out"=w340:errorcluster, "Values"=→"Sensor Value":bool[], "LINX Resource"=w341:T7)  [unwired: 6 in]
    n177 = call-poly <vilib>:"Servo Set Pulse Width.vi"("Error In"=w363, "Pulse Width (uS)"=w352, "Servo Channel"=w355, "LINX Resource"=w364) -> ("Error Out"=w360:errorcluster, "LINX Resource"=w361:T7)  [unwired: 6 in]
    n178 = Multiply(x="Servo Slider 1 Angle", y=u16 14) -> (x*y=w348:u16)
    n179 = call-poly <vilib>:"Digital Write.vi"("Error In"=w340, "Values"="Values", "DO Channels"=u8[] [24, 49, 51, 53], "LINX Resource"=w341) -> ("Error Out"=w332:errorcluster, "LINX Resource"=w333:T7)  [unwired: 6 in]
    n180 = call-poly <vilib>:"Servo Set Pulse Width.vi"("Error In"=w360, "Pulse Width (uS)"=w348, "Servo Channel"=w356, "LINX Resource"=w361) -> ("Error Out"=w358:errorcluster, "LINX Resource"=w359:T7)  [unwired: 6 in]
    n181 = Divide(x="Duty Cycle", y=100.0) -> (x/y=w343:dbl)
    n182 = Multiply(x="Servo Slider 2 Angle", y=u16 14) -> (x*y=w345:u16)
    n183 = call-poly <vilib>:"PWM Set Duty Cycle.vi"("Error In"=w332, "Duty Cycle (0-1)"=w343, "PWM Channel"="Speed Pin", "LINX Resource"=w333) -> ("Error Out"=w337:errorcluster, "LINX Resource"=w365:T7)  [unwired: 6 in]
    n184 = call-poly <vilib>:"Servo Set Pulse Width.vi"("Error In"=w358, "Pulse Width (uS)"=w345, "Servo Channel"=w357, "LINX Resource"=w359) -> ("Error Out"=w336:errorcluster, "LINX Resource"=w354:T7)  [unwired: 6 in]
    n185 = Compound Arithmetic op=OR(w337, w336, "STOP") -> (w369:bool)
  }
  n186 = Build Array(w6, w5, w4) -> (w7:u8[])
  n187 = call-poly <vilib>:"Servo Close.vi"("Error In"=w17, "Servo Channels"=w7, "LINX Resource"=w12) -> ("Error Out"=w13:errorcluster, "LINX Resource"=w14:T7)  [unwired: 7 in]
  n188 = call <vilib>:"Close.vi"("Error In"=w23, "LINX Resource"=w24) -> ()  [unwired: 9 in, 1 out]
  n189 = call <vilib>:"Close.vi"("Error In"=w13, "LINX Resource"=w14) -> ()  [unwired: 9 in, 1 out]
  n190 = call <vilib>:"Close.vi"("Error In"=w2, "LINX Resource"=w3) -> ()  [unwired: 9 in, 1 out]
